vi "Set Path.vi"(8 "error in (no error)":errorcluster, 10 "Measurement specfic paths":T1=enum."Harmonics", 11 "PathControl in":refnum<class "PathControl.lvclass">) -> (0 "error out":errorcluster, 3 "PathControl out":refnum<class "PathControl.lvclass">)   [LabVIEW 2020, in "PathControl.lvclass"]
uses:
  PathControl.lvclass
  Measurements Specific Paths.ctl
  PathControl.lvclass/PathControl.ctl
  Instruments/Path Switch/Path Switch.lvclass
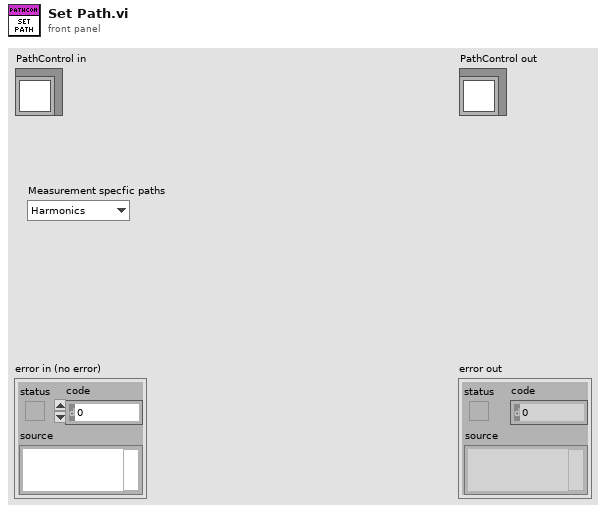
[diagram p1: front panel]
types:
  T1 = typedef "PathControl.lvclass/Measurements Specific Paths.ctl" = enum16{"No calibration", "Harmonics", "IMD", "S Parameter", "AM-AM", "MCCW-ACLR", "DC", "LCR", "Power Meter GUI", "RF Power"}
  T2 = cluster{"Name":string, "Path Frequency":dbl[], "Path Loss":dbl[]}[]
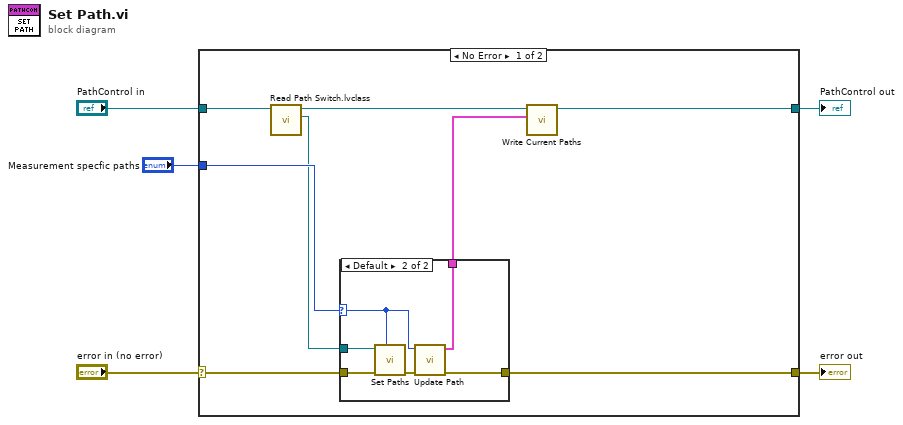
[diagram p0: block diagram]
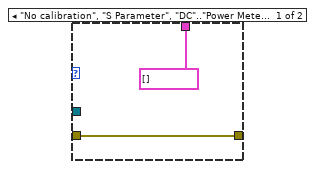
[diagram p2: hidden frame]
diagram:
  n1 = case shown="No Error" "error in (no error)" {
    selector: "error in (no error)" -> [w7 w23]
    tunnel: [w8 w23] -> w4
    tunnel: [w10 w22] -> w2
    tunnel: "PathControl in" -> [w13 w22]
    tunnel: "Measurement specfic paths" -> [w11 _]
    frame No Error {
      n2 = call "Read Path Switch.lvclass.vi"("PathControl in"=w13) -> ("Path Switch.lvclass"=w6:refnum<class "Path Switch.lvclass">, "PathControl out"=w12:refnum<class "PathControl.lvclass">)  [unwired: 9 in]
      n3 = case shown="Default" w11 {
        selector: w11 -> [_ w16]
        tunnel: [T2 [] ("Current Paths") w21] -> w9
        tunnel: [w14 w20] -> w8
        tunnel: w7 -> [w14 w19]
        tunnel: w6 -> [_ w18]
        frame "No calibration", "S Parameter", "DC".."Power Meter GUI" {
        }
        frame Default {
          n4 = call-dynamic "Set Paths.vi"("Measurement specfic paths"=w16, "error in (no error)"=w19, "Path Switch in"=w18) -> ("error out"=w17:errorcluster)  [unwired: 7 in, 1 out]
          n5 = call "Update Path.vi"("Error In"=w17, "Measurement specfic paths"=w16) -> ("Error Out"=w20:errorcluster, "Current Paths"=w21:T2)  [unwired: 8 in]
        }
      }
      n6 = call "Write Current Paths.vi"("Current Paths"=w9, "PathControl in"=w12) -> ("PathControl out"=w10:refnum<class "PathControl.lvclass">)  [unwired: 9 in]
    }
    frame Error {
    }
  }
  "error out" <- w4
  "PathControl out" <- w2
